vi "irrigationSystem.vi"() -> ()   [LabVIEW 2025]
uses:
  <vilib>/Instr/_visa.llb/VISA Configure Serial Port (Instr).vi
panel:
  out "shouldWater":bool
  out "Rotation":dbl(graph)
  out "Lux":dbl(graph)
  out "Humidity":dbl(graph)
  out "Temperature":dbl(graph)
  in  "stop":bool
  out "error out":errorcluster
  out "Debug":string
  in  "VISA resource name":refnum<visa-resource-name>
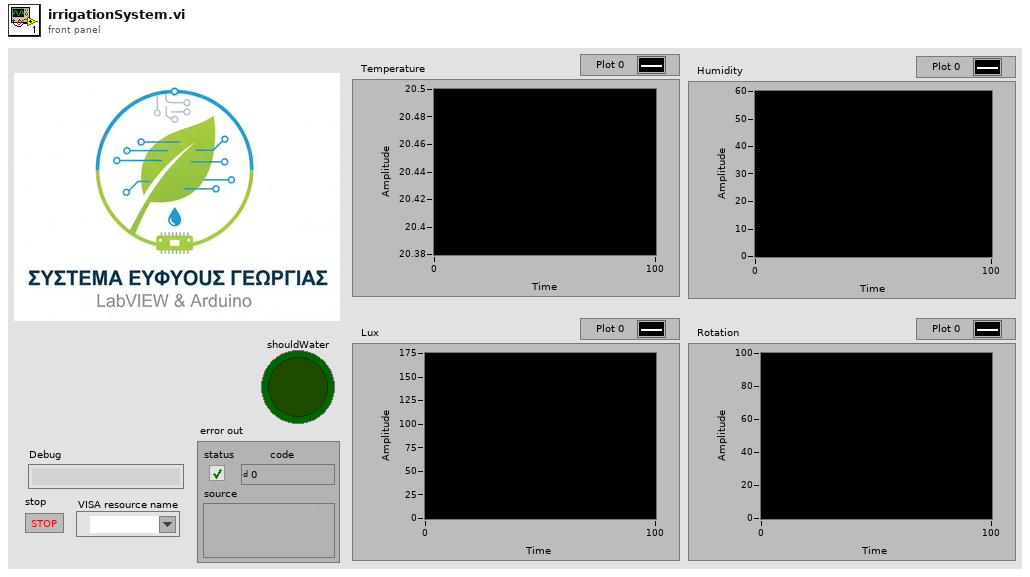
[diagram p1: front panel]
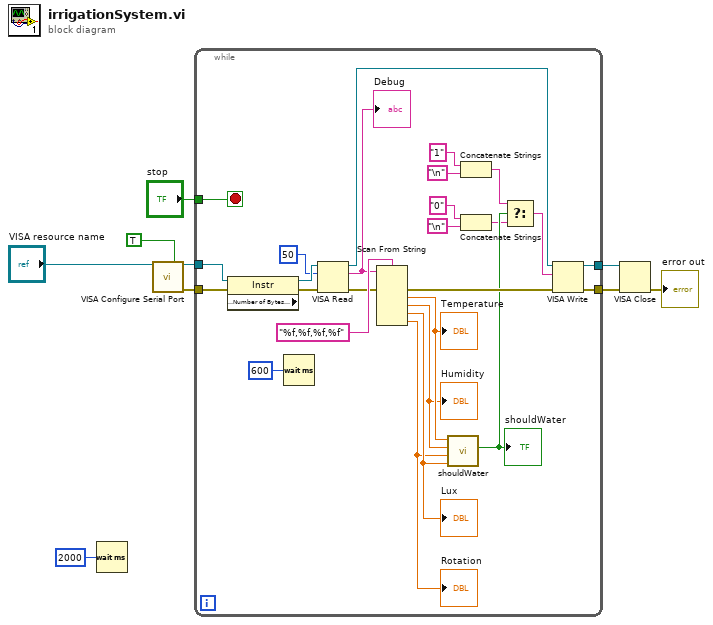
[diagram p0: block diagram]
diagram:
  n1 = Wait (ms)(milliseconds to wait=u32 2000) -> ()  [unwired: 1 out]
  n2 = call-poly "VISA Configure Serial Port"("VISA resource name"="VISA resource name", "Enable Termination\nChar (T)"=TRUE ("Enable Termination\nChar (T)")) -> ("VISA resource name out"=w8:refnum<visa-resource-name>, "error out"=w7:errorcluster)  [unwired: 12 in]
  n3 = while {
    tunnel: w8 -> [w35]
    tunnel: w7 -> [w31]
    tunnel: [w18] -> w5
    tunnel: "stop" -> [w26]
    tunnel: [w17] -> w2
    stop <- w26 stop-if-true
    n4 = property class="Instr" props=["Serial Settings:Number of Bytes at Serial Port"](reference=w35, error in=w31) -> (reference out=w34:refnum<visa-resource-name>, error out=w32:errorcluster)  [unwired: 1 out]
    n5 = Wait (ms)(milliseconds to wait=u32 600) -> ()  [unwired: 1 out]
    n6 = VISA Read(VISA resource name=w34, byte count=u32 50, error in (no error)=w32) -> (VISA resource name out=w25:refnum<visa-resource-name>, read buffer=w28:string, error out=w29:errorcluster)  [unwired: 1 out]
    "Debug" <- w28
    n7 = Scan From String(format string="%f,%f,%f,%f", input string=w28, error in=w29) -> (error out=w19:errorcluster, output 1=w24:dbl, output 2=w23:dbl, output 3=w22:dbl, output 4=w21:dbl)  [unwired: 5 in, 2 out]
    "Humidity" <- w23
    "Lux" <- w22
    "Temperature" <- w24
    "Rotation" <- w21
    n8 = call "shouldWater.vi"("lightLevel"=w22, "soilMoist"=w21, "airRH"=w23, "tempC"=w24) -> ("shouldWater"=w16:bool)  [unwired: 7 in]
    "shouldWater" <- w16
    n9 = Concatenate Strings("1", "\n") -> (w13:string)
    n10 = Concatenate Strings("0", "\n") -> (w10:string)
    n11 = Select(t=w13, s=w16, f=w10) -> (s? t:f=w20:string)
    n12 = VISA Write(VISA resource name=w25, write buffer=w20, error in (no error)=w19) -> (VISA resource name out=w17:refnum<visa-resource-name>, error out=w18:errorcluster)  [unwired: 1 out]
  }
  n13 = VISA Close(VISA resource name=w2, error in (no error)=w5) -> (error out=→"error out":errorcluster)
